vi "gfitsio-write-key-double.vi"(4 "units":string, 6 "comment":string, 7 "keyname":string, 8 "error in (no error)":errorcluster, 9 "value":dbl, 11 "gfits refnum":T1) -> (0 "error out":errorcluster, 3 "dup gfits refnum":T1)   [LabVIEW 2014, in "gfitsio.lvlib"]
doc: "Write a keyword of the appropriate data type into the current HDU. If the keyword already exists it will be overwritten. Otherwise a new keyword will be appended to the header."
uses:
  gfitsio.lvlib
  gfitsio-refnum.ctl
  cfitsio-datatypes.ctl
  gfitsio.dll
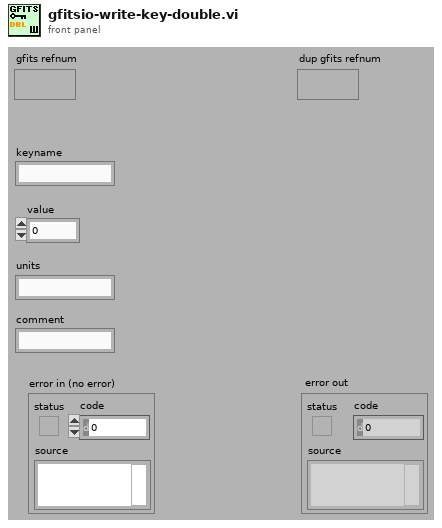
[diagram p1: front panel]
types:
  T1 = typedef "gfitsio.lvlib/gfitsio-refnum.ctl" = refnum<k1>
  T2 = typedef "gfitsio.lvlib/cfitsio-datatypes.ctl" = i32
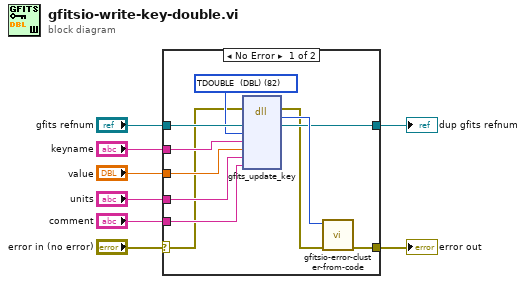
[diagram p0: block diagram]
diagram:
  n1 = case shown="No Error" "error in (no error)" {
    selector: "error in (no error)" -> [w10 w21]
    tunnel: [w18 w21] -> w4
    tunnel: "gfits refnum" -> [w16 w20]
    tunnel: [w17 w20] -> w7
    tunnel: "keyname" -> [w14 _]
    tunnel: "value" -> [w13 _]
    tunnel: "comment" -> [w12 _]
    tunnel: "units" -> [w11 _]
    frame No Error {
      w15 = T2 82 items=["TBIT"=1, "TBYTE  (U8)"=11, "TSBYTE  (I8)"=12, "TLOGICAL"=14, "TSTRING"=16, "TUSHORT  (U16)"=20, "TSHORT  (I16)"=21, "TUINT"=31, "TULONG  (U32)"=40, "TLONG  (I32)"=41, "TFLOAT  (SGL)"=42, "TLONGLONG  (I64)"=81, "TDOUBLE  (DBL)"=82, "TCOMPLEX  (CSG)"=83, "TDOUBLECOMPLEX  (CDB)"=163] ("cfitsio datatype")
      n2 = dll-call lib="D:/optics_and_proj_related_stuff/labview_codes/gfitsio/gfitsio.dll" fn="gfits_update_key"(error in=w10, "gfits refnum"=w16, "datatype"=w15, "keyname"=w14, "value"=w13, "unit"=w11, "comment"=w12) -> (error out=w9:errorcluster, w19:i32, "gfits refnum"=w17:T1)  [unwired: 7 in, 1 out]
      n3 = call "gfitsio-error-cluster-from-code.vi"("error in (no error)"=w9, "error code"=w19) -> ("error out"=w18:errorcluster)  [unwired: 9 out]
    }
    frame Error {
    }
  }
  "error out" <- w4
  "dup gfits refnum" <- w7
